vi "7L21-qsinit.vi"(1 "Qs (e)":T1) -> (0 "Qs (s)":T1)   [LabVIEW 2010, in "lv_07.lvlib"]
doc: "Si le risque est à 0, il est initialisé à 5% (0,05)"
uses:
  lv_07.lvlib
  c_Qs_.ctl
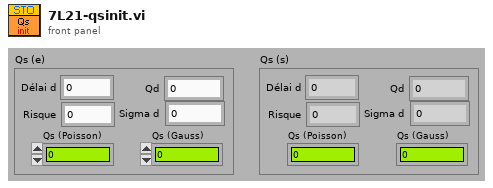
[diagram p1: front panel]
types:
  T1 = typedef "lv_07.lvlib/c_Qs_.ctl" = cluster{"Sigma d":dbl, "Qs (Gauss)":dbl, "Qs (Poisson)":dbl, "Qd":dbl, "Délai d":dbl, "Risque":dbl}
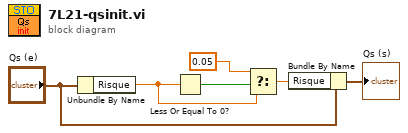
[diagram p0: block diagram]
diagram:
  n1 = Unbundle By Name("Qs (e)") -> ("Risque"=w3:dbl)
  n2 = Less Or Equal To 0?(x=w3) -> (x <= 0?=w1:bool)
  n3 = Select(t=0.05 ("cas vrai"), s=w1, f=w3) -> (s? t:f=w4:dbl)
  n4 = Bundle By Name(cluster="Qs (e)", "Risque"=w4) -> (→"Qs (s)":T1)
